vi "DAC Save Results.vi"(8 "error in":errorcluster, 9 "Log Details?":bool, 10 "tdms file":refnum<k34>, 11 "DAC TC Temperature in":refnum<class "DAC TC Temp CryoSep.lvclass">) -> (0 "error out":errorcluster)   [LabVIEW 2019, in "DAC.lvlib" / "DAC TC Temp CryoSep.lvclass"]
uses:
  DAC TC Temp CryoSep.lvclass
  C:/Users/krio/Documents/LV_Projects/test-stand/App/DAC/DAC.lvclass
  DAC.lvclass/DAC.ctl
  DAC TC Temp CryoSep.lvclass/DAC TC Temp CryoSep.ctl
  DAC.lvclass
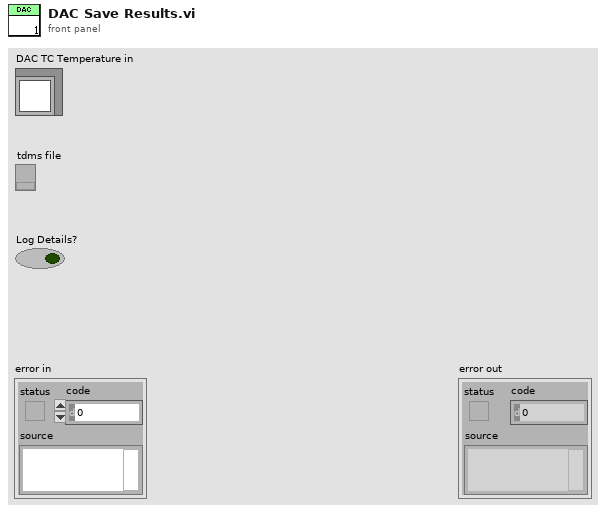
[diagram p1: front panel]
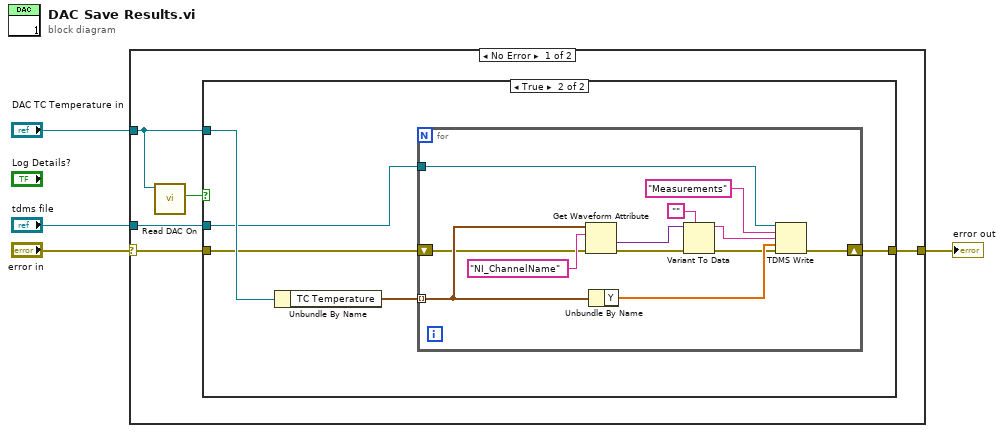
[diagram p0: block diagram]
diagram:
  n1 = case shown="No Error" "error in" {
    selector: "error in" -> [w6 w28]
    tunnel: "DAC TC Temperature in" -> [w9 _]
    tunnel: "tdms file" -> [w7 _]
    tunnel: [w5 w28] -> w1
    frame No Error {
      n2 = call "Read DAC On.vi"("DAC in"=w9) -> ("DAC On"=w8:bool)  [unwired: 8 in, 2 out]
      n3 = case shown="True" w8 {
        tunnel: w9 -> [_ w15]
        tunnel: w7 -> [_ w14]
        tunnel: w6 -> [w10 w12]
        tunnel: [w10 w11] -> w5
        frame False {
        }
        frame True {
          n4 = Unbundle By Name(w15) -> ("TC Temperature"=w13:waveform(dbl)[])
          n5 = for {
            tunnel: w14 -> [w27]
            tunnel: w13 -> [w20] mode=indexing
            shift-right: [w16] -> w11
            shift-left: w12 -> [w19]
            n6 = Get Waveform Attribute(4:w19, 6:"NI_ChannelName" ("name"), 7:w20) -> (0:w18:errorcluster, 1:w25:variant)  [unwired: 1 in, 2 out]
            n7 = Unbundle By Name(w20) -> ("Y"=w22:dbl[])
            n8 = Variant To Data(error in=w18, type="", Variant=w25) -> (data=w21:string, error out=w17:errorcluster)
            n9 = TDMS Write(0:w27, 5:"Measurements" ("group name in (Untitled)"), 7:w21, 9:w22, 11:w17) -> (15:w16:errorcluster)  [unwired: 1 in, 3 out]
          }
        }
      }
    }
    frame Error {
    }
  }
  "error out" <- w1
